vi "Only_Alphanumeric_Character (SubVI).vi"(8 "error in (no error)":errorcluster, 11 "Character":i16) -> (0 "error out (no error)":errorcluster, 3 "Discard character taped":bool)   [LabVIEW 2011]
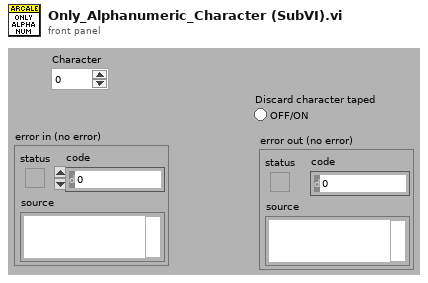
[diagram p1: front panel]
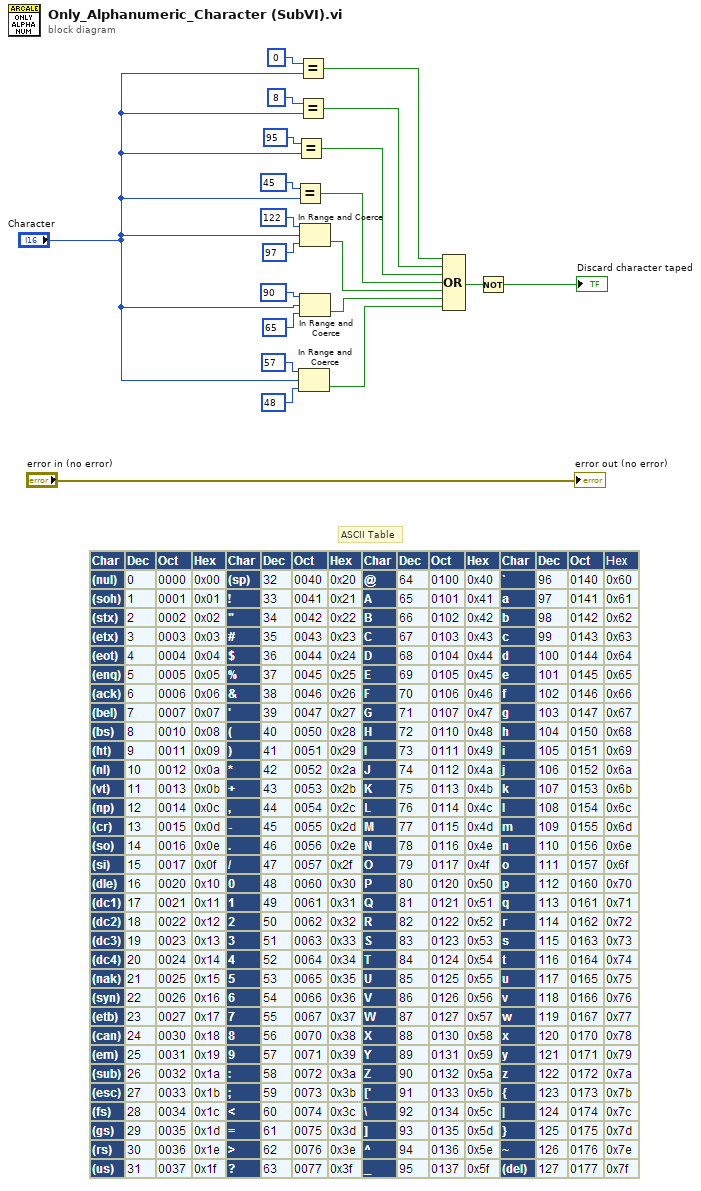
[diagram p0: block diagram]
diagram:
  # "ASCII Table"
  n1 = Equal?(x=i16 45, y="Character") -> (x = y?=w12:bool)
  n2 = Equal?(x=i16 95, y="Character") -> (x = y?=w13:bool)
  n3 = Equal?(x=i16 0, y="Character") -> (x = y?=w1:bool)
  n4 = Equal?(x=i16 8, y="Character") -> (x = y?=w5:bool)
  n5 = In Range and Coerce(upper limit=i16 57, x="Character", lower limit=i16 48 ("upper limit")) -> (In Range?=w9:bool)  [unwired: 1 out]
  n6 = In Range and Coerce(upper limit=i16 122, x="Character", lower limit=i16 97 ("upper limit")) -> (In Range?=w11:bool)  [unwired: 1 out]
  n7 = In Range and Coerce(upper limit=i16 90, x="Character", lower limit=i16 65 ("upper limit")) -> (In Range?=w10:bool)  [unwired: 1 out]
  n8 = Compound Arithmetic op=OR(w1, w5, w13, w12, w11, w10, w9) -> (w4:bool)
  n9 = Not(x=w4) -> (.not. x?=→"Discard character taped":bool)
  "error out (no error)" <- "error in (no error)"
